vi "Check Game Done.vi"(8 "error in (no error)":errorcluster, 10 "Won":bool, 11 "SB App in":refnum<class "SB App.lvclass">) -> (0 "error out":errorcluster, 2 "Done?":bool, 3 "SB App out":refnum<class "SB App.lvclass">)   [LabVIEW 2020, in "SB App.lvlib" / "SB App.lvclass"]
uses:
  SB App.lvclass
  SB App.lvclass/SB App.ctl
  SquareBattle/Game/Game.lvclass
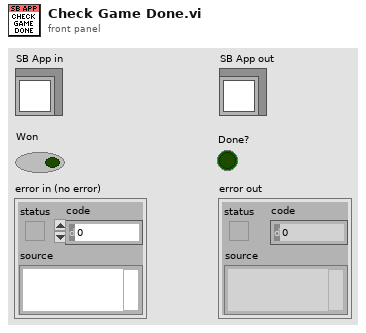
[diagram p1: front panel]
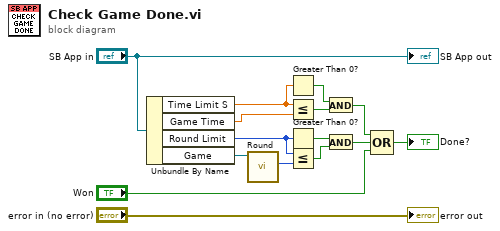
[diagram p0: block diagram]
diagram:
  n1 = Unbundle By Name("SB App in") -> ("Time Limit S"=w8:dbl, "Game Time"=w11:dbl, "Round Limit"=w7:u32, "Game"=w13:refnum<class "Game.lvclass">)
  n2 = call "Round.vi"("Game in"=w13) -> ("Round"=w12:u32)  [unwired: 8 in, 2 out]
  n3 = Greater Than 0?(x=w8) -> (x > 0?=w3:bool)
  n4 = Less Or Equal?(x=w8, y=w11) -> (x <= y?=w4:bool)
  n5 = Greater Than 0?(x=w7) -> (x > 0?=w6:bool)
  n6 = Less Or Equal?(x=w7, y=w12) -> (x <= y?=w5:bool)
  n7 = And(x=w3, y=w4) -> (x .and. y?=w1:bool)
  n8 = And(x=w6, y=w5) -> (x .and. y?=w2:bool)
  n9 = Compound Arithmetic op=OR(w1, w2, "Won") -> (→"Done?":bool)
  "error out" <- "error in (no error)"
  "SB App out" <- "SB App in"
